vi "Read write template.vi"() -> ()   [LabVIEW 2012]
doc: "This VI shows how to use Network Streams to read data from one process and write to another."
uses:
  Datatype B.ctl
  Datatype A.ctl
panel:
  in  "stop":bool
  out "Data A read":T1
  in  "Array of B Data":T2[](array[typedef])
  in  "Data A writer endpoint URL":string="//localhost/Data A Writer name"
  # "This example demonstrates how Network Streams could be used in a robotics application.  Examine the block diagrams of the example VIs to see the implementation.\n\nTo use this architecture, modify the data types according to what you need and update the URL's to point to the correct endpoint (changing localhost to the appropriate IP address, for example).  Then run the following VI's in any order:\nRead write template.vi\nWrite template.vi\nRead template.vi\n\nSee the readme.html for more help using this architecture with an RT Target."
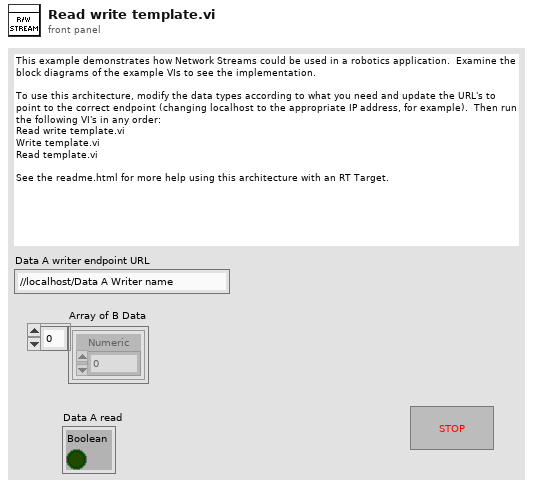
[diagram p1: front panel]
types:
  T1 = typedef "Datatype A.ctl" = cluster{"Boolean":bool}
  T2 = typedef "Datatype B.ctl" = cluster{"Numeric":dbl}
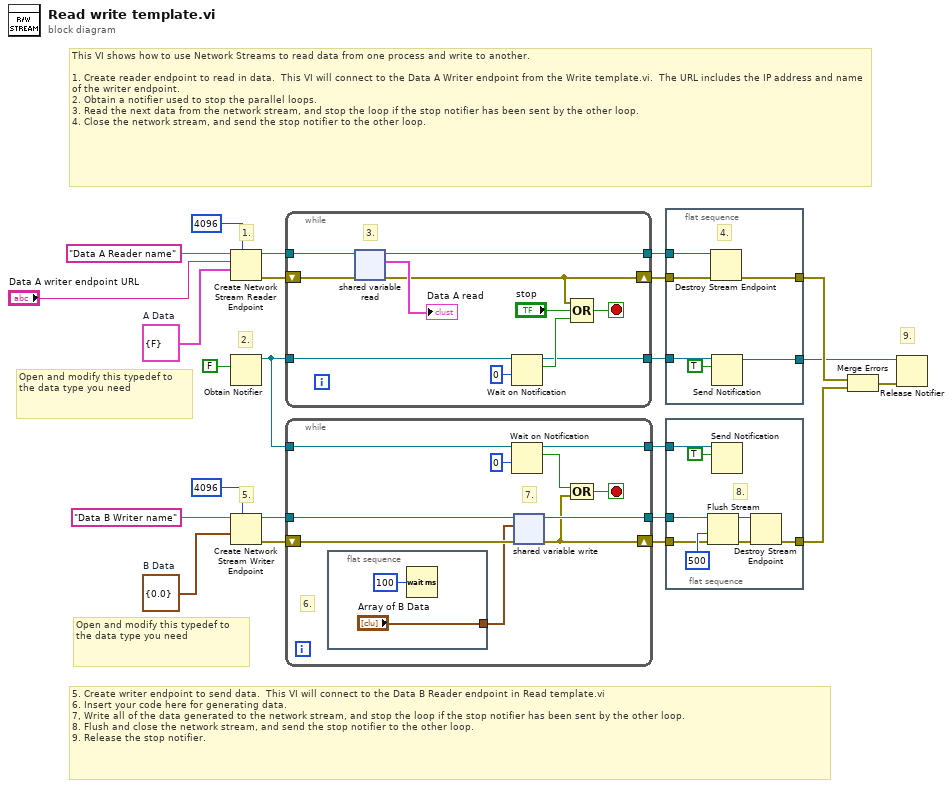
[diagram p0: block diagram]
diagram:
  w12 = T1 {"Boolean"=FALSE}  # A Data
  w13 = T2 {"Numeric"=0.0}  # B Data
  # "9."
  # "2."
  # "Open and modify this typedef to the data type you need"
  # "Open and modify this typedef to the data type you need"
  # "5."
  # "5. Create writer endpoint to send data.  This VI will connect to the Data B Reader endpoint in Read template.vi\n6. Insert your code here for generating data.\n7, Write all of the data generated to the network stream, and stop the loop if the stop notifier has been sent by the other loop.\n8. Flush and close the network stream, and send the stop notifier to the other loop.\n9. Release the stop notifier."
  # "1."
  # "This VI shows how to use Network Streams to read data from one process and write to another.  \n\n1. Create reader endpoint to read in data.  This VI will connect to the Data A Writer endpoint from the Write template.vi.  The URL includes the IP address and name of the writer endpoint.\n2. Obtain a notifier used to stop the parallel loops.\n3. Read the next data from the network stream, and stop the loop if the stop notifier has been sent by the other loop.\n4. Close the network stream, and send the stop notifier to the other loop."
  n1 = Create Network Stream Reader Endpoint(7:4096 ("reader buffer size"), 9:w12, 10:"Data A writer endpoint URL", 11:"Data A Reader name" ("reader name")) -> (0:w20:errorcluster, 3:w21:refnum<k21>)  [unwired: 3 in]
  n2 = Obtain Notifier(notification data type=FALSE) -> (notifier out=w9:refnum<notifier>)  [unwired: 3 in, 2 out]
  n3 = Create Network Stream Writer Endpoint(7:4096 ("writer buffer size"), 9:w13, 11:"Data B Writer name" ("writer name")) -> (0:w15:errorcluster, 3:w16:refnum<k21>)  [unwired: 4 in]
  n4 = while {
    tunnel: w21 -> [w34]
    tunnel: [w32] -> w19
    tunnel: w9 -> [w28]
    tunnel: [w24] -> w8
    shift-right: [w25] -> w18
    shift-left: w20 -> [w33]
    stop <- w29 stop-if-true
    # "3."
    n5 = shared-variable-read(w34, w33) -> (w32:refnum<k21>, w25:errorcluster, →"Data A read":T1)  [unwired: 1 in, 1 out]
    n6 = Wait on Notification(notifier=w28, timeout in ms (-1)=0) -> (notifier out=w24:refnum<notifier>, notification=w26:bool)  [unwired: 2 in, 2 out]
    n7 = Compound Arithmetic op=OR(w25, "stop", w26) -> (w29:bool)
  }
  n8 = while {
    tunnel: w16 -> [w44]
    tunnel: [w43] -> w11
    tunnel: w9 -> [w39]
    tunnel: [w35] -> w7
    shift-right: [w38] -> w14
    shift-left: w15 -> [w42]
    stop <- w36 stop-if-true
    # "7."
    # "6."
    n9 = flat-sequence {
      tunnel: ["Array of B Data"] -> w41
      frame #0 {
        n10 = Wait (ms)(milliseconds to wait=u32 100) -> ()  [unwired: 1 out]
      }
    }
    n11 = Wait on Notification(notifier=w39, timeout in ms (-1)=0) -> (notifier out=w35:refnum<notifier>, notification=w37:bool)  [unwired: 2 in, 2 out]
    n12 = shared-variable-write(w44, w42, w41) -> (w43:refnum<k21>, w38:errorcluster)  [unwired: 1 in, 1 out]
    n13 = Compound Arithmetic op=OR(w37, w38) -> (w36:bool)
  }
  n14 = flat-sequence {
    tunnel: w19 -> [w52]
    tunnel: w18 -> [w51]
    tunnel: w8 -> [w50]
    tunnel: [w48] -> w6
    tunnel: [w47] -> w4
    frame #0 {
      # "4."
      n15 = Destroy Stream Endpoint(8:w51, 11:w52) -> (0:w48:errorcluster)
      n16 = Send Notification(notification=TRUE, notifier=w50) -> (notifier out=w47:refnum<notifier>)  [unwired: 1 in, 1 out]
    }
  }
  n17 = flat-sequence {
    tunnel: w14 -> [w57]
    tunnel: w11 -> [w56]
    tunnel: w7 -> [w54]
    tunnel: [w53] -> w5
    frame #0 {
      # "8."
      n18 = Flush Stream(8:w57, 9:500 ("timeout in ms (-1)"), 11:w56) -> (0:w60:errorcluster, 3:w59:refnum<k21>)  [unwired: 1 in, 1 out]
      n19 = Send Notification(notification=TRUE, notifier=w54) -> ()  [unwired: 1 in, 2 out]
      n20 = Destroy Stream Endpoint(8:w60, 11:w59) -> (0:w53:errorcluster)
    }
  }
  n21 = Merge Errors(w6, w5) -> (w3:errorcluster)
  n22 = Release Notifier(notifier=w4, error in (no error)=w3) -> ()  [unwired: 1 in, 3 out]
